vi "CRYUpdate Buttons.vi"   [LabVIEW 2013]
uses:
  Global/CRYCurve Library Global.vi
panel:
  # "Update Buttons of Curve Library"
types:
  T1 = enum8{"Enabled", "Disabled", "Disabled and Grayed Out"}
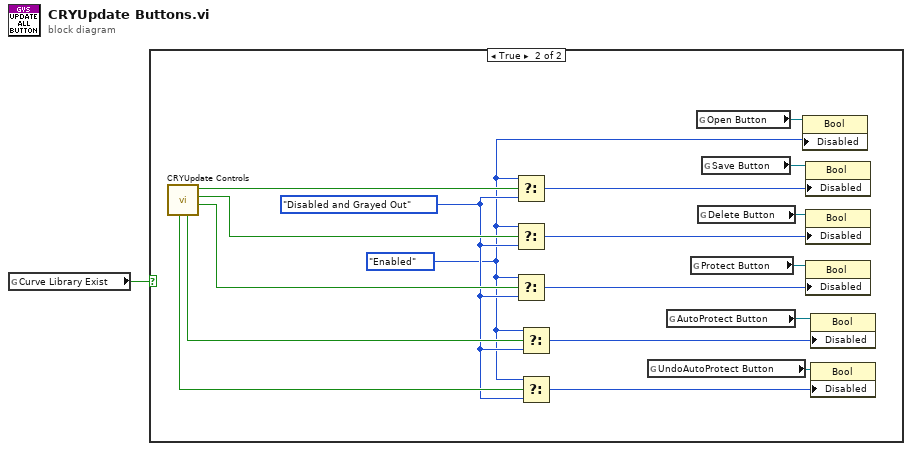
[diagram p0: block diagram]
diagram:
  n1 = global read "CRYCurve Library Global.vi" "Curve Library Exist"() -> (w1:bool)
  n2 = case shown="True" w1 {
    frame False {
    }
    frame True {
      w4 = T1."Disabled and Grayed Out" ("Disabled")
      w3 = T1."Enabled" ("Disabled")
      n3 = call "CRYUpdate Controls.vi"() -> ("Protect?"=w14:bool, "Delete/Rename?"=w13:bool, "Save/Export?"=w6:bool, "AutoProtect?"=w8:bool, "UndoAutoProtect?"=w7:bool)  [unwired: 7 out]
      n4 = Select(t=w3, s=w6, f=w4) -> (s? t:f=w2:T1)
      n5 = Select(t=w3, s=w13, f=w4) -> (s? t:f=w15:T1)
      n6 = Select(t=w3, s=w14, f=w4) -> (s? t:f=w16:T1)
      n7 = Select(t=w3, s=w8, f=w4) -> (s? t:f=w11:T1)
      n8 = Select(t=w3, s=w7, f=w4) -> (s? t:f=w12:T1)
      n9 = global read "CRYCurve Library Global.vi" "UndoAutoProtect Button"() -> (w10:refnum<vi>)
      n10 = global read "CRYCurve Library Global.vi" "AutoProtect Button"() -> (w9:refnum<vi>)
      n11 = global read "CRYCurve Library Global.vi" "Protect Button"() -> (w17:refnum<vi>)
      n12 = global read "CRYCurve Library Global.vi" "Open Button"() -> (w5:refnum<vi>)
      n13 = global read "CRYCurve Library Global.vi" "Delete Button"() -> (w18:refnum<vi>)
      n14 = global read "CRYCurve Library Global.vi" "Save Button"() -> (w19:refnum<vi>)
      n15 = property class="Bool"(reference=w5, "Disabled"=w3) -> ()  [unwired: 1 in, 2 out]
      n16 = property class="Bool"(reference=w19, "Disabled"=w2) -> ()  [unwired: 1 in, 2 out]
      n17 = property class="Bool"(reference=w18, "Disabled"=w15) -> ()  [unwired: 1 in, 2 out]
      n18 = property class="Bool"(reference=w17, "Disabled"=w16) -> ()  [unwired: 1 in, 2 out]
      n19 = property class="Bool"(reference=w9, "Disabled"=w11) -> ()  [unwired: 1 in, 2 out]
      n20 = property class="Bool"(reference=w10, "Disabled"=w12) -> ()  [unwired: 1 in, 2 out]
    }
  }
